vi "Back Grabber Control Read.vi"(1 "Controller State":T1 {"POV" items=["None"=-1, "POV Up"=0, "POV Up Right"=1, "POV Right"=2, "POV Down Right"=3, "POV Down"=4, "POV Down Left"=5, "POV Left"=6, "POV Up Left"=7]}) -> (0 "State out":i16)   [LabVIEW 2010, in "4150_RingItUp_State.lvrbt"]
uses:
  4150_RingItUp_State/4150_RingItUp_State.lvrbt
  <vilib>/FTC/FTC ControllerState.ctl
  <vilib>/FTC/FTC POVState.ctl
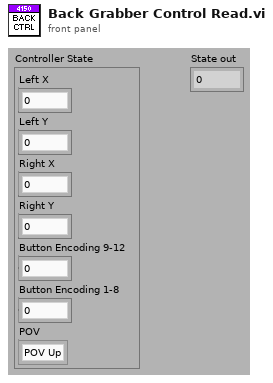
[diagram p1: front panel]
types:
  T1 = typedef "FTC ControllerState.ctl" = cluster{"Left X":i8, "Left Y":i8, "Right X":i8, "Right Y":i8, "Button Encoding 9-12":u8, "Button Encoding 1-8":u8, "POV":T2}
  T2 = typedef "FTC POVState.ctl" = i8
  T3 = typedef "FTC ButtonState.ctl" = cluster{"Button 1":bool, "Button 2":bool, "Button 3":bool, "Button 4":bool, "Button 5":bool, "Button 6":bool, "Button 7":bool, "Button 8":bool, "Button 9":bool, "Button 10":bool, "Button 11":bool, "Button 12":bool, "POV":T2}
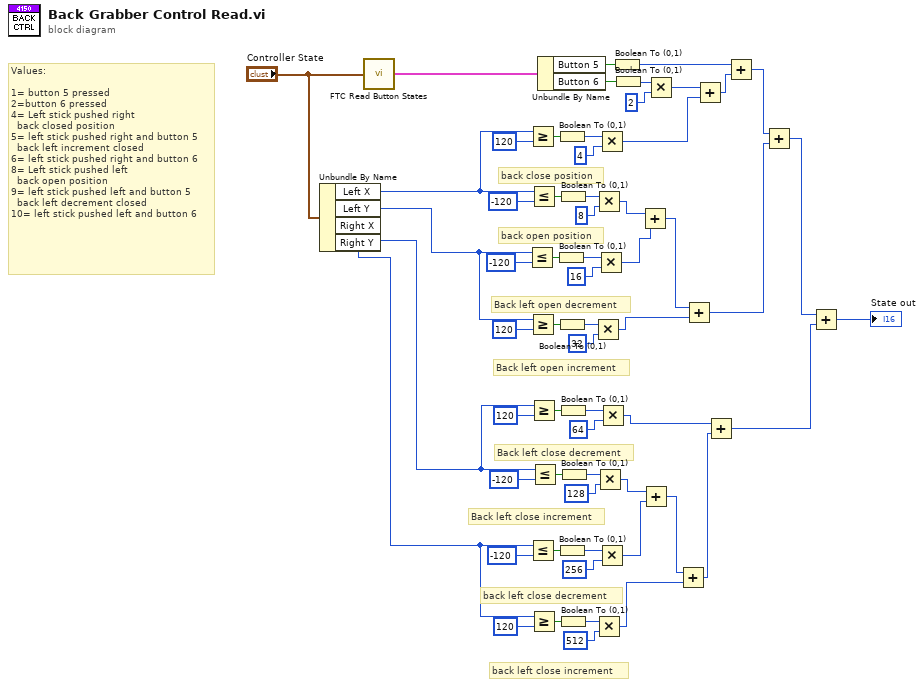
[diagram p0: block diagram]
diagram:
  # "Values:\n\n1= button 5 pressed\n2=button 6 pressed\n4= Left stick pushed right\n  back closed position\n5= left stick pushed right and button 5\n  back left increment closed\n6= left stick pushed right and button 6\n8= Left stick pushed left\n  back open position\n9= left stick pushed left and button 5\n  back left decrement closed\n10= left stick pushed left and button 6"
  # "Back left open increment"
  # "Back left open decrement"
  # "back open position"
  # "back left close decrement"
  # "Back left close decrement"
  # "Back left close increment"
  # "back left close increment"
  # "back close position"
  n1 = Unbundle By Name("Controller State") -> ("Left X"=w43:i8, "Left Y"=w33:i8, "Right X"=w7:i8, "Right Y"=w6:i8)
  n2 = call <vilib>:"FTC Read Button States.vi"("Controller State"="Controller State") -> ("Button States"=w46:T3)  [unwired: 2 in, 1 out]
  n3 = Less Or Equal?(x=w33, y=i8 -120) -> (x <= y?=w36:bool)
  n4 = Greater Or Equal?(x=w43, y=i8 120) -> (x >= y?=w48:bool)
  n5 = Greater Or Equal?(x=w33, y=i8 120) -> (x >= y?=w37:bool)
  n6 = Less Or Equal?(x=w6, y=i8 -120) -> (x <= y?=w21:bool)
  n7 = Less Or Equal?(x=w43, y=i8 -120) -> (x <= y?=w49:bool)
  n8 = Greater Or Equal?(x=w7, y=i8 120) -> (x >= y?=w13:bool)
  n9 = Greater Or Equal?(x=w6, y=i8 120) -> (x >= y?=w20:bool)
  n10 = Less Or Equal?(x=w7, y=i8 -120) -> (x <= y?=w12:bool)
  n11 = Unbundle By Name(w46) -> ("Button 5"=w47:bool, "Button 6"=w56:bool)
  n12 = Boolean To (0,1)(Boolean=w36) -> (0, 1=w38:i16)
  n13 = Boolean To (0,1)(Boolean=w48) -> (0, 1=w50:i16)
  n14 = Boolean To (0,1)(Boolean=w37) -> (0, 1=w40:i16)
  n15 = Boolean To (0,1)(Boolean=w21) -> (0, 1=w19:i16)
  n16 = Boolean To (0,1)(Boolean=w49) -> (0, 1=w54:i16)
  n17 = Boolean To (0,1)(Boolean=w13) -> (0, 1=w11:i16)
  n18 = Boolean To (0,1)(Boolean=w20) -> (0, 1=w17:i16)
  n19 = Boolean To (0,1)(Boolean=w12) -> (0, 1=w9:i16)
  n20 = Multiply(x=w40, y=i16 32) -> (x*y=w29:i16)
  n21 = Multiply(x=w54, y=i16 8) -> (x*y=w32:i16)
  n22 = Multiply(x=w17, y=i16 512) -> (x*y=w27:i16)
  n23 = Multiply(x=w9, y=i16 128) -> (x*y=w24:i16)
  n24 = Multiply(x=w38, y=i16 16) -> (x*y=w31:i16)
  n25 = Multiply(x=w50, y=i16 4) -> (x*y=w61:i16)
  n26 = Multiply(x=w19, y=i16 256) -> (x*y=w25:i16)
  n27 = Multiply(x=w11, y=i16 64) -> (x*y=w5:i16)
  n28 = Boolean To (0,1)(Boolean=w47) -> (0, 1=w51:i16)
  n29 = Boolean To (0,1)(Boolean=w56) -> (0, 1=w57:i16)
  n30 = Add(x=w32, y=w31) -> (x+y=w30:i16)
  n31 = Add(x=w24, y=w25) -> (x+y=w26:i16)
  n32 = Multiply(x=w57, y=i16 2) -> (x*y=w60:i16)
  n33 = Add(x=w26, y=w27) -> (x+y=w4:i16)
  n34 = Add(x=w30, y=w29) -> (x+y=w28:i16)
  n35 = Add(x=w60, y=w61) -> (x+y=w59:i16)
  n36 = Add(x=w5, y=w4) -> (x+y=w3:i16)
  n37 = Add(x=w51, y=w59) -> (x+y=w52:i16)
  n38 = Add(x=w52, y=w28) -> (x+y=w1:i16)
  n39 = Add(x=w1, y=w3) -> (x+y=→"State out":i16)
